vi "Leak Detector LabView.vi"() -> ()   [LabVIEW 2025]
uses:
  <vilib>/Instr/_visa.llb/VISA Configure Serial Port (Instr).vi
  <vilib>/Utility/file.llb/Write Delimited Spreadsheet (string).vi
panel:
  out "Check ongoing":bool
  out "File Path":path
  out "Leak Rate XY Graph":cluster{dbl[], dbl[]}(graph)
  out "Factor":bool
  out "Decreased":bool
  out "Factor":bool
  out "Decreasing":bool
  out "Stabilising":bool
  out "Sample Rate (Seconds)":dbl
  out "Test Duration (seconds)":dbl
  out "Stabilised":bool
  out "Time":timestamp[](array[timestamp])
  in  "Stabilisation Check":bool
  out "Index":dbl[](array[numeric])
  out "Leak Rate":dbl[](array[numeric])
  out "Stabilisation error":bool
  out "File Save Error":errorcluster
  out "Leak Rate Waveform":dbl(graph)
  out "P2 Waveform":dbl(graph)
  in  "Stop on error":bool
  out "Read Bytes":u32
  out "P2 (mbar)":string
  out "Write Bytes":u32
  out "Read Bytes":u32
  out "Write Bytes":u32
  out "Leak Rate (sccs)":string
  out "Available resource names":string[](array[string])
  out "Connected?":bool
  out "Error":errorcluster
  in  "VISA resource name":refnum<visa-resource-name>
  in  "Max Pressure (bar)":u32
  in  "Min Pressure  (bar)":u32
  in  "Loop Rate (ms)":u32
  in  "Save File":bool
  out "Pressure Transducer Waveform":dbl(graph)
  out "Connected?":bool
  in  "Read Names":string[](array[string])=["AIN0", "FIO2"]
  out "Pressure - raw voltage (v)":dbl[](array[numeric]) format="%.6f"
  in  "stop":bool
  out "Error String":string
  out "ConnectionType":i32
  out "Device Type":i32
  out "Error":errorcluster
  # "LabJack"
  # "Use this button to stop only"
  # "Leak Detector"
  # "Leak Rate"
  # "P2"
  # "Condition Current Status"
  # "Condition Met"
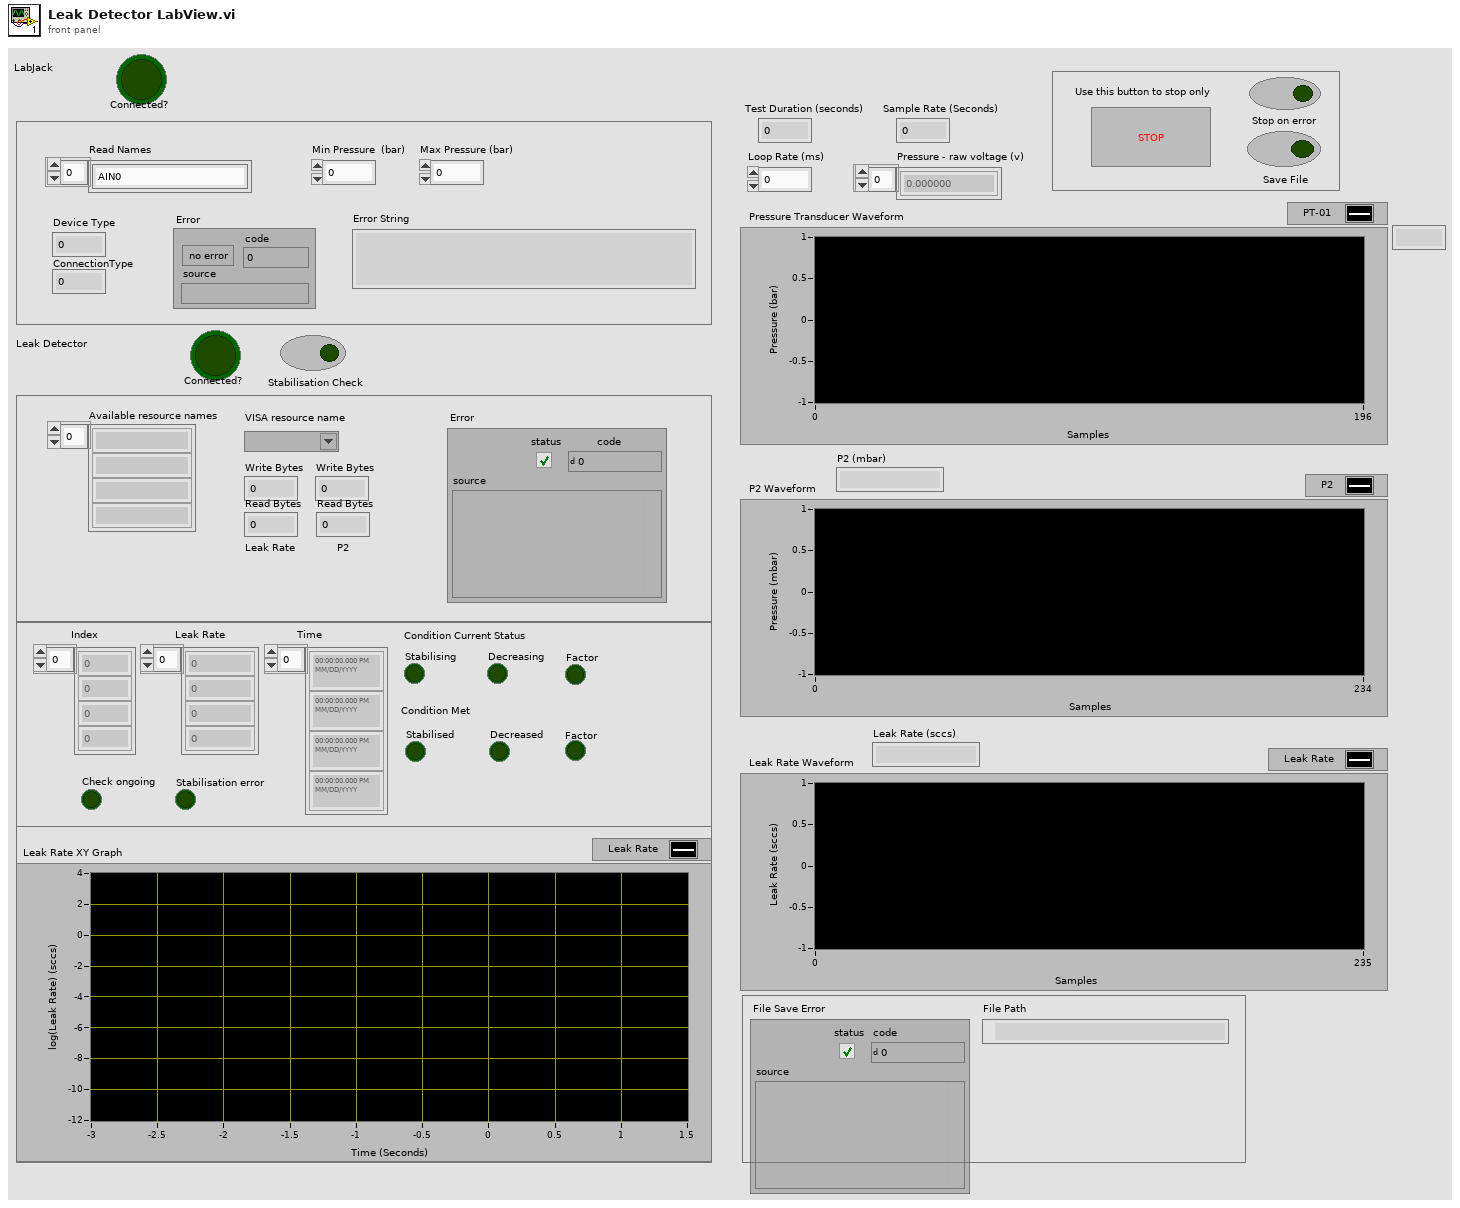
[diagram p1: front panel]
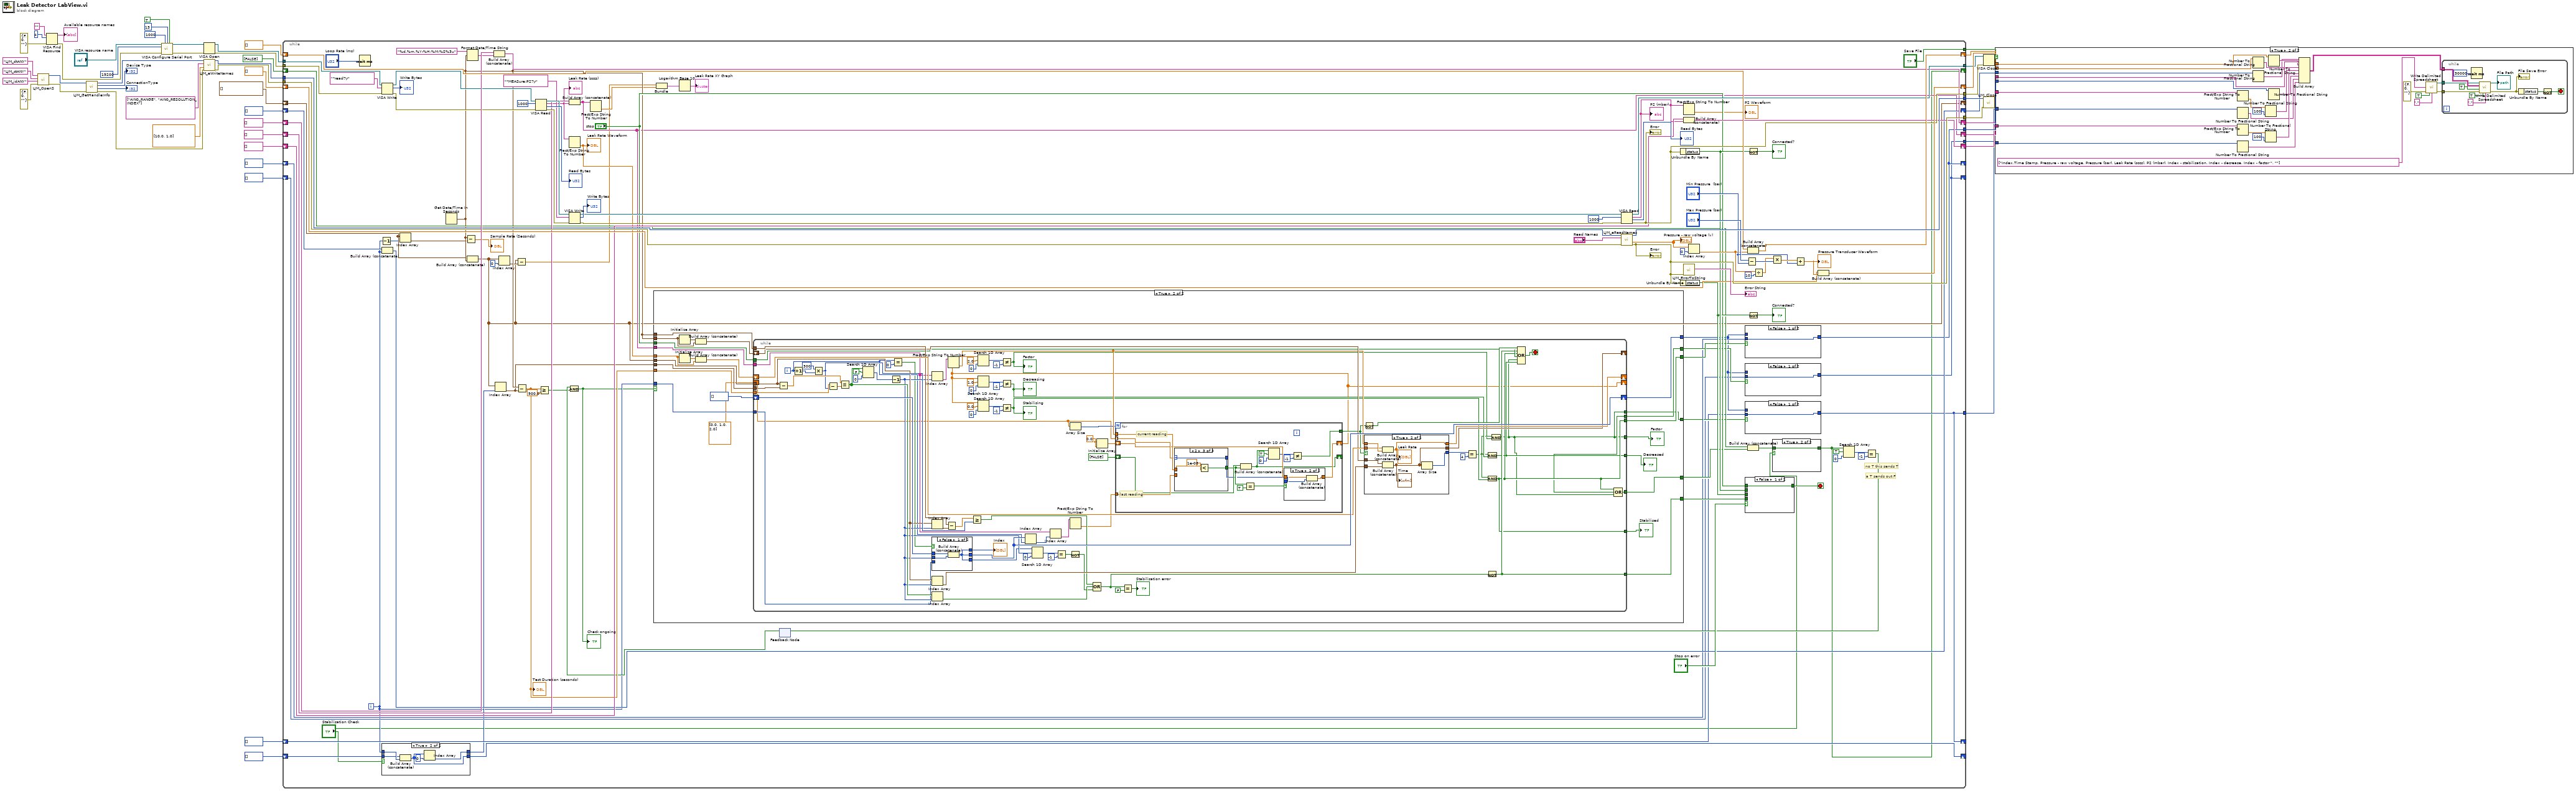
[diagram p0: block diagram]
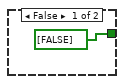
[diagram p3: hidden frame]
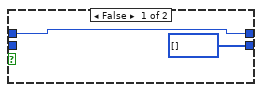
[diagram p4: hidden frame]
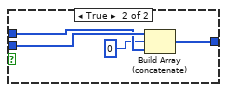
[diagram p5: hidden frame]
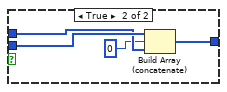
[diagram p6: hidden frame]
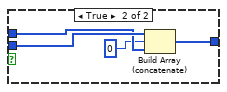
[diagram p7: hidden frame]
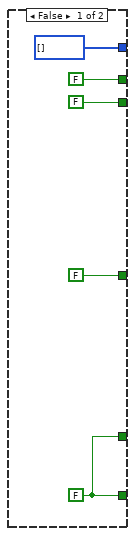
[diagram p8: hidden frame]
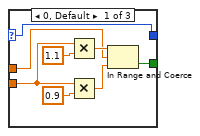
[diagram p10: hidden frame]
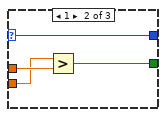
[diagram p11: hidden frame]
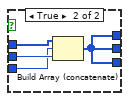
[diagram p12: hidden frame]
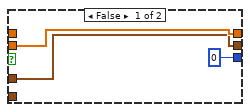
[diagram p13: hidden frame]
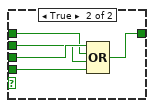
[diagram p14: hidden frame]
diagram:
  n1 = call <vilib>:"LJM_OpenS.vi"("error in"=errorcluster {"status"=FALSE, "code"=0, "source"=""} ("error in (no error)"), "Identifier"="LJM_idANY", "ConnectionType"="LJM_ctANY", "DeviceType"="LJM_dtANY") -> ("error out"=w53:errorcluster, "Handle"=w52:i32)  [unwired: 6 in]
  n2 = VISA Find Resource(8:errorcluster {"status"=FALSE, "code"=0, "source"=""} ("error in (no error)"), 10:4 ("code"), 11:"" ("source")) -> (0:w29:errorcluster, 3:→"Available resource names":string[])  [unwired: 1 out]
  n3 = call <vilib>:"LJM_GetHandleInfo.vi"("error in"=w53, "Handle In"=w52) -> ("error out"=w43:errorcluster, "ConnectionType"=→"ConnectionType":i32, "DeviceType"=→"Device Type":i32, "Handle Out"=w47:i32)  [unwired: 2 in, 4 out]
  n4 = call-poly "VISA Configure Serial Port"("VISA resource name"="VISA resource name", "timeout (10sec)"=u32 1000, "termination char\n(0xA = '\\n' = LF)"=13, "Enable Termination\nChar (T)"=TRUE, "baud rate (9600)"=19200 ("code"), "error in (no error)"=w29) -> ("VISA resource name out"=w33:refnum<visa-resource-name>, "error out"=w35:errorcluster)  [unwired: 4 in, 4 out]
  n5 = VISA Open(error in (no error)=w35, VISA resource name=w33) -> (VISA resource name=w32:refnum<visa-resource-name>, error out=w34:errorcluster)  [unwired: 3 in]
  n6 = call <vilib>:"LJM_eWriteNames.vi"("Handle In"=w47, "aNames"=string[] ["AIN0_RANGE", "AIN0_RESOLUTION_INDEX"], "aValuesIn"=dbl[] [10.0, 1.0], "error in"=w43) -> ("Handle Out"=w20:i32, "error out"=w48:errorcluster)  [unwired: 9 in, 1 out]
  n7 = while {
    tunnel: w48 -> [w147]
    tunnel: [w154] -> w50
    tunnel: [w157] -> w49
    shift-right: [w152] -> w41
    shift-left: dbl[] [] -> [w153]
    shift-right: [w108] -> w6
    shift-left: string[] [] -> [w151]
    shift-right: [w140] -> w38
    shift-left: dbl[] [] -> [w139]
    tunnel: ["Save File"] -> w37
    tunnel: w32 -> [w134]
    tunnel: w34 -> [w133]
    tunnel: [w117] -> w36
    tunnel: [w116] -> w21
    shift-right: [w81] -> w7
    shift-left: string[] [] -> [w114]
    shift-right: [w113] -> w8
    shift-left: string[] [] -> [w112]
    tunnel: w20 -> [w109]
    shift-right: [w60] -> _
    shift-left: timestamp[] [] -> [w85]
    shift-right: [w104] -> w9
    shift-left: i32[] [] -> [w105]
    shift-right: [w58] -> _
    shift-left: bool[] [FALSE] -> [w98]
    tunnel: [w92] -> w10
    shift-right: [w92] -> _
    shift-left: i32[] [] -> [w74]
    tunnel: [w68] -> w5
    tunnel: [w66] -> w4
    shift-right: [w68] -> _
    shift-left: i32[] [] -> [w69]
    shift-right: [w66] -> _
    shift-left: i32[] [] -> [w67]
    shift-right: [w61] -> _
    shift-left: i32[] [] -> [w59]
    i -> [w62]
    stop <- w101 stop-if-true
    # "a T sends out F"
    # "no T this sends T"
    n8 = Wait (ms)(milliseconds to wait="Loop Rate (ms)") -> ()  [unwired: 1 out]
    n9 = Decrement(x=w62) -> (x-1=w82:i32)
    n10 = VISA Write(VISA resource name=w134, write buffer="*read?\r", error in (no error)=w133) -> (VISA resource name out=w128:refnum<visa-resource-name>, return count=→"Write Bytes":u32, error out=w129:errorcluster)
    n11 = Build Array (concatenate)(w105, w62) -> (w104:i32[])
    n12 = case shown="True" "Stabilisation Check" {
      tunnel: [w162 w163] -> w63
      tunnel: w62 -> [w162 w167]
      tunnel: w59 -> [_ w166]
      tunnel: [i32[] [] w165] -> w61
      frame False {
      }
      frame True {
        n13 = Build Array (concatenate)(w166, w167) -> (w165:i32[])
        n14 = Index Array(array=w165, index=0) -> (element=w163:i32)
      }
    }
    n15 = Index Array(array=w85, index=w82) -> (element=w84:timestamp)
    n16 = Get Date/Time In Seconds() -> (seconds since 1Jan1904=w86:timestamp)
    n17 = Subtract(x=w86, y=w84) -> (x-y=→"Sample Rate (Seconds)":dbl)
    n18 = Format Date/Time String(time format string (%c)="%d.%m.%Y-%H:%M:%S%3u", seconds (now)=w86) -> (date/time string=w148:string)  [unwired: 1 in]
    n19 = Build Array (concatenate)(w85, w86) -> (w60:timestamp[])
    n20 = Build Array (concatenate)(w151, w148) -> (w108:string[])
    n21 = Index Array(array=w60, index=w63) -> (element=w64:timestamp)
    n22 = Index Array(array=w60, index=0) -> (element=w79:timestamp)
    n23 = Subtract(x=w60, y=w79) -> (x-y=w77:dbl[])
    n24 = Subtract(x=w86, y=w64) -> (x-y=w106:dbl)
    "Test Duration (seconds)" <- w106
    n25 = VISA Read(VISA resource name=w128, byte count=u32 1000 ("timeout (10sec)"), error in (no error)=w129) -> (VISA resource name out=w123:refnum<visa-resource-name>, read buffer=w91:string, return count=→"Read Bytes":u32, error out=w124:errorcluster)
    "Leak Rate (sccs)" <- w91
    n26 = Greater Or Equal?(x=w106, y=900.0 ("element")) -> (x >= y?=w65:bool)
    n27 = Build Array (concatenate)(w114, w91) -> (w81:string[])
    n28 = Fract/Exp String To Number(string=w91) -> (number=w90:dbl)  [unwired: 3 in, 1 out]
    "Leak Rate Waveform" <- w90
    n29 = VISA Write(VISA resource name=w123, write buffer="*MEASure:P2?\r", error in (no error)=w124) -> (VISA resource name out=w119:refnum<visa-resource-name>, return count=→"Write Bytes":u32, error out=w120:errorcluster)
    n30 = Fract/Exp String To Number(string=w81) -> (number=w78:dbl[])  [unwired: 3 in, 1 out]
    n31 = Bundle(w77, w78) -> (w71:cluster{dbl[], dbl[]})  [unwired: 1 in]
    n32 = Logarithm Base 10(1:w71) -> (0:→"Leak Rate XY Graph":cluster{dbl[], dbl[]})
    n33 = feedback #1() -> (w87:bool)  [unwired: 1 in]
    n34 = Compound Arithmetic op=AND(w87, w65) -> (w56:bool)
    "Check ongoing" <- w56
    n35 = case shown="True" w56 {
      tunnel: w60 -> [_ w211]
      tunnel: w86 -> [_ w210]
      tunnel: w81 -> [_ w202]
      tunnel: w106 -> [_ w209]
      tunnel: [i32[] [] w208] -> w73
      tunnel: [w187 w207] -> w103
      tunnel: [w187 w192] -> w99
      tunnel: "stop" -> [_ w206]
      tunnel: w64 -> [_ w205]
      tunnel: w62 -> [_ w203]
      tunnel: w86 -> [_ w196]
      tunnel: w90 -> [_ w198]
      tunnel: [FALSE w195] -> w76
      tunnel: [FALSE w194] -> w75
      tunnel: [FALSE w193] -> w72
      frame False {
        w187 = FALSE
      }
      frame True {
        n36 = Initialize Array(w196) -> (w197:timestamp[])  [unwired: 1 in]
        n37 = Initialize Array(w198) -> (w199:dbl[])  [unwired: 1 in]
        n38 = Build Array (concatenate)(w197, w196) -> (w200:timestamp[])
        n39 = Build Array (concatenate)(w199, w198) -> (w201:dbl[])
        n40 = while {
          tunnel: w211 -> [w264]
          tunnel: w210 -> [w275]
          tunnel: w202 -> [w240]
          shift-right: [w281] -> w208
          shift-left: i32[] [] -> [w283]
          shift-right: [w279] -> _
          shift-left: w201 -> [w278]
          tunnel: w209 -> [w276]
          tunnel: [w259] -> w207
          shift-right: [w261] -> _
          shift-left: w200 -> [w262]
          tunnel: w206 -> [w260]
          tunnel: w205 -> [w258]
          tunnel: w203 -> [w247]
          tunnel: [w216] -> w195
          tunnel: [w215] -> w194
          tunnel: [w214] -> w193
          tunnel: [w217] -> w192
          tunnel: [w216] -> w191
          tunnel: [w215] -> w190
          tunnel: [w214] -> w189
          shift-right: [w212] -> _
          shift-left: dbl[] [0.0, 1.0, 2.0] ("aValuesIn") -> [w213]
          i -> [w241]
          stop <- w265 stop-if-true
          w236 = 0.0
          n41 = Subtract(x=w264, y=w258) -> (x-y=w274:dbl[])
          n42 = Increment(x=w241) -> (x+1=w285:i32)
          n43 = Multiply(x=u32 300 ("y"), y=w285) -> (x*y=w267:u32)
          n44 = Subtract(x=w276, y=w267) -> (x-y=w273:dbl)
          n45 = Less Or Equal?(x=w274, y=w273) -> (x <= y?=w269:bool[])
          n46 = Search 1D Array(1D array=w269, element=FALSE, start index (0)=0 ("index of element")) -> (index of element=w268:i32)
          n47 = Decrement(x=w268) -> (x-1=w256:i32)
          n48 = Equal?(x=w241, y=0) -> (x = y?=w237:bool)
          n49 = Index Array(array=w240, index=w256) -> (element=w246:string)
          n50 = Index Array(array=w264, index=w256) -> (element=w270:timestamp)
          n51 = case shown="False" w237 {
            tunnel: [w326 w330] -> w281
            tunnel: w283 -> [w328 w332]
            tunnel: [w326 w330] -> w277
            tunnel: w256 -> [w327 w331]
            tunnel: [w326 w330] -> w255
            tunnel: w247 -> [_ w329]
            frame False {
              n52 = Build Array (concatenate)(w328, w327) -> (w326:i32[])
            }
            frame True {
              n53 = Build Array (concatenate)(w332, w329, w331) -> (w330:i32[])
            }
          }
          "Index" <- w277
          n54 = Index Array(array=w264, index=w256) -> (element=w263:timestamp)
          n55 = Index Array(array=w269, index=w256) -> (element=w250:bool)
          n56 = Subtract(x=w275, y=w270) -> (x-y=w289:dbl)
          n57 = Fract/Exp String To Number(string=w246) -> (number=w242:dbl)  [unwired: 3 in, 1 out]
          n58 = Greater Or Equal?(x=w289, y=w267) -> (x >= y?=w251:bool)
          n59 = Index Array(array=w281, index=w241) -> (element=w280:i32)
          n60 = Search 1D Array(1D array=w255, element=w256, start index (0)=0 ("index of element")) -> (index of element=w254:i32)
          n61 = Index Array(array=w240, index=w280) -> (element=w245:string)
          n62 = Equal?(x=w254, y=-1) -> (x = y?=w252:bool)
          n63 = Not(x=w252) -> (.not. x?=w249:bool)
          n64 = Array Size(array=w213) -> (size(s)=w239:i32)
          n65 = Fract/Exp String To Number(string=w245) -> (number=w243:dbl)  [unwired: 3 in, 1 out]
          n66 = Compound Arithmetic op=OR(w251, w250, w249) -> (w248:bool)
          n67 = Initialize Array(w236, w236) -> (w238:dbl[])
          n68 = for {
            N: w239 -> [_]
            tunnel: w243 -> [w305]
            tunnel: w242 -> [w304]
            tunnel: w213 -> [w303] mode=indexing
            shift-right: [w291] -> _
            shift-left: bool[] [FALSE] -> [w298]
            tunnel: [w293] -> w221
            shift-right: [w299] -> w212
            shift-left: w238 -> [w300]
            # "current reading"
            # "last reading"
            n69 = case shown="2" w303 {
              selector: w303 -> [w310 w318 w322]
              tunnel: w305 -> [w313 w320 _]
              tunnel: w304 -> [w312 w321 w324]
              tunnel: [w311 w319 w325] -> w297
              tunnel: [w310 w318 w322] -> w290
              frame 0, Default {
                n70 = Multiply(x=w313, y=1.1 ("x*y")) -> (x*y=w317:dbl)
                n71 = Multiply(x=w313, y=0.9 ("x*y")) -> (x*y=w316:dbl)
                n72 = In Range and Coerce(upper limit=w317, x=w312, lower limit=w316) -> (In Range?=w311:bool)  [unwired: 1 out]
              }
              frame 1 {
                n73 = Greater?(x=w320, y=w321) -> (0:w319:bool)
              }
              frame 2 {
                n74 = Less?(x=w324, y=1e-08) -> (x < y?=w325:bool)
              }
            }
            n75 = Build Array (concatenate)(w298, w297) -> (w291:bool[])
            n76 = Equal?(x=w297, y=TRUE) -> (x = y?=w301:bool)
            n77 = Search 1D Array(1D array=w291, element=TRUE, start index (0)=0 ("index of element")) -> (index of element=w295:i32)
            n78 = case shown="True" w301 {
              tunnel: w290 -> [_ w307]
              tunnel: w300 -> [w306 w309]
              tunnel: [w306 w308] -> w299
              frame False {
              }
              frame True {
                n79 = Build Array (concatenate)(w309, w307) -> (w308:dbl[])
              }
            }
            n80 = Not Equal?(x=w295, y=-1 ("index of element")) -> (x != y?=w293:bool)
          }
          n81 = Search 1D Array(1D array=w212, element=2.0, start index (0)=0) -> (index of element=w225:i32)
          n82 = Search 1D Array(1D array=w212, element=1.0, start index (0)=0) -> (index of element=w226:i32)
          n83 = Search 1D Array(1D array=w212, element=0.0, start index (0)=0) -> (index of element=w229:i32)
          n84 = Not Equal?(x=w225, y=-1) -> (x != y?=w218:bool)
          "Factor" <- w218
          n85 = Not Equal?(x=w226, y=-1) -> (x != y?=w220:bool)
          "Decreasing" <- w220
          n86 = Not Equal?(x=w229, y=-1) -> (x != y?=w222:bool)
          "Stabilising" <- w222
          n87 = Equal?(x=w248, y=FALSE) -> (x = y?=→"Stabilisation error":bool)
          n88 = Not(x=w221) -> (.not. x?=w266:bool)
          n89 = case shown="True" w221 {
            tunnel: w242 -> [_ w342]
            tunnel: [w335 w340] -> w279
            tunnel: w278 -> [w335 w341]
            tunnel: w263 -> [_ w338]
            tunnel: w262 -> [w334 w339]
            tunnel: [w334 w337] -> w261
            tunnel: [0 w336] -> w244
            frame False {
            }
            frame True {
              n90 = Build Array (concatenate)(w341, w342) -> (w340:dbl[])
              "Leak Rate" <- w340
              n91 = Build Array (concatenate)(w339, w338) -> (w337:timestamp[])
              "Time" <- w337
              n92 = Array Size(array=w337) -> (size(s)=w336:i32)
            }
          }
          n93 = Equal?(x=w244, y=4) -> (x = y?=w219:bool)
          n94 = Not(x=w248) -> (.not. x?=w259:bool)
          n95 = And(x=w219, y=w220) -> (x .and. y?=w215:bool)
          n96 = And(x=w219, y=w222) -> (x .and. y?=w216:bool)
          n97 = And(x=w219, y=w218) -> (x .and. y?=w214:bool)
          n98 = Compound Arithmetic op=OR(w266, w259, w216, w260, w214, w215) -> (w265:bool)
          n99 = Compound Arithmetic op=OR(w216, w215, w214) -> (w217:bool)
        }
        "Stabilised" <- w191
        "Decreased" <- w190
        "Factor" <- w189
      }
    }
    n100 = VISA Read(VISA resource name=w119, byte count=u32 1000 ("timeout (10sec)"), error in (no error)=w120) -> (VISA resource name out=w116:refnum<visa-resource-name>, read buffer=w89:string, return count=→"Read Bytes":u32, error out=w117:errorcluster)
    "Error" <- w117
    "P2 (mbar)" <- w89
    n101 = call <vilib>:"LJM_eReadNames.vi"("Handle In"=w109, "aNames"="Read Names", "error in"=w147) -> ("Handle Out"=w157:i32, "aValuesOut"=w150:dbl[], "error out"=w154:errorcluster)  [unwired: 9 in, 1 out]
    "Pressure - raw voltage (v)" <- w150
    "Error" <- w154
    n102 = Unbundle By Name(w117) -> ("status"=w131:bool)
    n103 = Unbundle By Name(w154) -> ("status"=w111:bool)
    n104 = Fract/Exp String To Number(string=w89) -> (number=→"P2 Waveform":dbl)  [unwired: 3 in, 1 out]
    n105 = Build Array (concatenate)(w112, w89) -> (w113:string[])
    n106 = call <vilib>:"LJM_ErrorToString.vi"("error in"=w154) -> ("String"=→"Error String":string)  [unwired: 10 in]
    n107 = Index Array(array=w150, index=0) -> (element=w138:dbl)
    n108 = case shown="False" w76 {
      tunnel: w73 -> [_ w180]
      tunnel: w74 -> [w178 w182]
      tunnel: [w178 w181] -> w92
      frame False {
      }
      frame True {
        n109 = Build Array (concatenate)(w182, 0, w180) -> (w181:i32[])
      }
    }
    n110 = case shown="False" w75 {
      tunnel: w73 -> [_ w175]
      tunnel: w69 -> [w173 w177]
      tunnel: [w173 w176] -> w68
      frame False {
      }
      frame True {
        n111 = Build Array (concatenate)(w177, 0, w175) -> (w176:i32[])
      }
    }
    n112 = case shown="False" w72 {
      tunnel: w73 -> [_ w170]
      tunnel: w67 -> [w168 w172]
      tunnel: [w168 w171] -> w66
      frame False {
      }
      frame True {
        n113 = Build Array (concatenate)(w172, 0, w170) -> (w171:i32[])
      }
    }
    n114 = case shown="False" "Stop on error" {
      tunnel: "stop" -> [w343 w347]
      tunnel: w131 -> [_ w346]
      tunnel: w111 -> [_ w348]
      tunnel: [w343 w345] -> w101
      tunnel: w103 -> [_ w344]
      frame False {
      }
      frame True {
        n115 = Compound Arithmetic op=OR(w348, w347, w346, w344) -> (w345:bool)
      }
    }
    n116 = Subtract(x="Max Pressure (bar)", y="Min Pressure  (bar)") -> (x-y=w144:u32)
    n117 = Not(x=w131) -> (.not. x?=→"Connected?":bool)
    n118 = Build Array (concatenate)(w153, w138) -> (w152:dbl[])
    n119 = Not(x=w111) -> (.not. x?=→"Connected?":bool)
    n120 = Build Array (concatenate)(w98, w99) -> (w57:bool[])
    n121 = Divide(x=w138, y=10) -> (x/y=w136:dbl)
    n122 = Multiply(x=w136, y=w144) -> (x*y=w143:dbl)
    n123 = case shown="True" "Stabilisation Check" {
      tunnel: [bool[] [FALSE] w160] -> w58
      tunnel: w57 -> [_ w160]
      frame False {
      }
      frame True {
      }
    }
    n124 = Add(x=w143, y="Min Pressure  (bar)") -> (x+y=w141:dbl)
    "Pressure Transducer Waveform" <- w141
    n125 = Build Array (concatenate)(w139, w141) -> (w140:dbl[])
    n126 = Search 1D Array(1D array=w58, element=TRUE, start index (0)=0 ("index of element")) -> (index of element=w95:i32)
    n127 = Equal?(x=w95, y=-1 ("index of element")) -> (x = y?=w93:bool)
    n128 = feedback-in #1(w93) -> ()
  }
  n129 = VISA Close(VISA resource name=w21, error in (no error)=w36) -> ()  [unwired: 1 out]
  n130 = call <vilib>:"LJM_Close.vi"("error in"=w50, "Handle"=w49) -> ()  [unwired: 9 in, 1 out]
  n131 = case shown="True" w37 {
    tunnel: w6 -> [_ w376]
    tunnel: w41 -> [_ w374]
    tunnel: w38 -> [_ w372]
    tunnel: w7 -> [_ w366]
    tunnel: w8 -> [_ w365]
    tunnel: w10 -> [_ w369]
    tunnel: w9 -> [_ w368]
    tunnel: w5 -> [_ w356]
    tunnel: w4 -> [_ w355]
    frame False {
    }
    frame True {
      n132 = Fract/Exp String To Number(string=w366) -> (number=w363:dbl[])  [unwired: 3 in, 1 out]
      n133 = Number To Fractional String(number=w356) -> (F-format string=w358:string[])  [unwired: 3 in]
      n134 = Fract/Exp String To Number(string=w365) -> (number=w364:dbl[])  [unwired: 3 in, 1 out]
      n135 = Number To Fractional String(number=w355) -> (F-format string=w357:string[])  [unwired: 3 in]
      n136 = Number To Fractional String(number=w372) -> (F-format string=w371:string[])  [unwired: 3 in]
      n137 = Number To Fractional String(number=w368) -> (F-format string=w367:string[])  [unwired: 3 in]
      n138 = Number To Fractional String(number=w363, precision (6)=i16 100) -> (F-format string=w362:string[])  [unwired: 2 in]
      n139 = Number To Fractional String(number=w364, precision (6)=i16 100 ("width (-)")) -> (F-format string=w361:string[])  [unwired: 2 in]
      n140 = Number To Fractional String(number=w374) -> (F-format string=w373:string[])  [unwired: 3 in]
      n141 = Number To Fractional String(number=w369) -> (F-format string=w370:string[])  [unwired: 3 in]
      n142 = Build Array(w367, w376, w373, w371, w362, w361, w370, w358, w357) -> (w375:string[][])
      n143 = call-poly <vilib>:"Write Delimited Spreadsheet.vi"("1D data"=string[] ["Index,Time Stamp, Pressure - raw voltage, Pressure (bar), Leak Rate (sccs), P2 (mbar), Index - stabilisation, Index - decrease, Index - factor ", ""] ("aNames"), "error in (no error)"=errorcluster {"status"=FALSE, "code"=0, "source"=""}, "transpose? (no:F)"=TRUE, "delimiter (\\t)"="," ("delimiter (\\t)")) -> ("new file path (Not A Path if cancelled)"=w354:path, "error out"=w349:errorcluster)  [unwired: 10 in]
      n144 = while {
        tunnel: w375 -> [w386]
        tunnel: w354 -> [w379]
        tunnel: w349 -> [w378]
        stop <- w382 stop-if-true
        n145 = Wait (ms)(milliseconds to wait=u32 30000) -> ()  [unwired: 1 out]
        n146 = call-poly <vilib>:"Write Delimited Spreadsheet.vi"("file path (dialog if empty)"=w379, "2D data"=w386, "append to file? (new file:F)"=TRUE ("transpose? (no:F)"), "error in (no error)"=w378, "transpose? (no:F)"=TRUE, "delimiter (\\t)"="," ("delimiter (\\t)")) -> ("new file path (Not A Path if cancelled)"=→"File Path":path, "error out"=w384:errorcluster)  [unwired: 8 in]
        "File Save Error" <- w384
        n147 = Unbundle By Name(w384) -> ("status"=w383:bool)
        n148 = Not(x=w383) -> (.not. x?=w382:bool)
      }
    }
  }
